vi "Stroker Wizard.vi"(1 "Stroker Wizard L1":u16, 2 "Stroker Wizard L2":u16, 11 "error in (no error)":errorcluster) -> ()   [LabVIEW 2011]
uses:
  Analog Var Disp 0 sif.ctl
  Status indicator Black Small.ctl
  Controls/Tristate/Tristate Valve state.ctl
  Controls/Slips Type Radio.ctl
  Tool/Variable List Tool Analog.ctl
  Application Structure/Options/Action GFV Settings.ctl
  Tool/Stroker/def/Tool specific commands.ctl
  Application Structure/Options/Options PageID.ctl
  Measurments Handling/Common/Variable List Common Digital.ctl
  Measurments Handling/Status Digitalish.ctl
  Tool/Variable List Tool Digital.ctl
  Application Structure/QSM State List.ctl
  emi Lib/System 01/0 - General/App/Loop control 2/Private/_emi_SMLoop Control Single.vi
  emi Lib/System 01/0 - General/App/Loop control 2/Private/_emi_ SMLoop start condition.vi
  emi Lib/System 01/0 - General/App/Loop control 2/Private/_emi_ SMLoop Error Check.vi
  emi Lib/Basic/0 - General/Error/emi_Is Error.vi
  emi Lib/System 01/0 - General/App/Loop control 2/Private/_emi_SMLoop Register new.vi
  emi Lib/System 01/0 - General/S&E reporting/emi_Send S&E Error message.vi
  emi Lib/Basic/0 - General/Error/emi_ Is Error state.vi
  emi Lib/System 01/0 - General/emi_Read System ID.vi
  emi Lib/System 01/0 - General/App/Loop control/Private/_emi_GFV Loop Running.vi
  emi Lib/System 01/0 - General/App/Loop control 2/Private/_emi_ SMLoop Restart Counter.vi
  emi Lib/System 01/0 - General/App/Loop control/Private/_emi_GFV stop a loop so it can reset.vi
  emi Lib/System 01/0 - General/App/Loop control 2/Private/_emi_ SMLoop Restart.vi
  emi Lib/System 01/0 - General/App/Loop control/Private/_emi_GFV Loop Linking.vi
  emi Lib/System 01/0 - General/App/Loop control/Private/_emi_GFV Loop Enable.vi
  emi Lib/System 01/0 - General/App/Private/_emi_GFV App Close.vi
  emi Lib/System 01/0 - General/Private/_emi_GFV System ID.vi
  emi Lib/System 01/0 - General/S&E reporting/Private/_emi_S&E Q Generator.vi
panel:
  in  "Tab Control":enum32{"Waiting", "Wizard", "Timeout"}(tab)
  out "Waiting Lights":T1
  in  "Close":bool
  in  "Size":T2=enum."338 MRS"
  out "Voltage Down Hole":T3={"Value"=nan, "Unit"="", "Status"=0} caption="Voltage Downhole(PCP)" {"Value" format="%#.1f"}
  out "St Anchor":T5 caption="Anchor"
  out "St Solonoid State Stroker":T5 caption="Direction"
  out "St Solonoid State Master":T5 caption="Stroker Enabled"
  in  "Go to default pos":bool
  out "Anchor behavior":string
  out "Stroker behavior":string
  out "Stroker force limit":string caption="tonne"
  in  "Timeout Close":bool
  # "Waiting for Telemetry to start"
  # "Stroker Wizard"
  # "Default Settings"
  # "Slips"
  # "Solenoid positions"
  # "Telemetry Timeout!"
  # "Telemetry failed to start. Voltage will be reset."
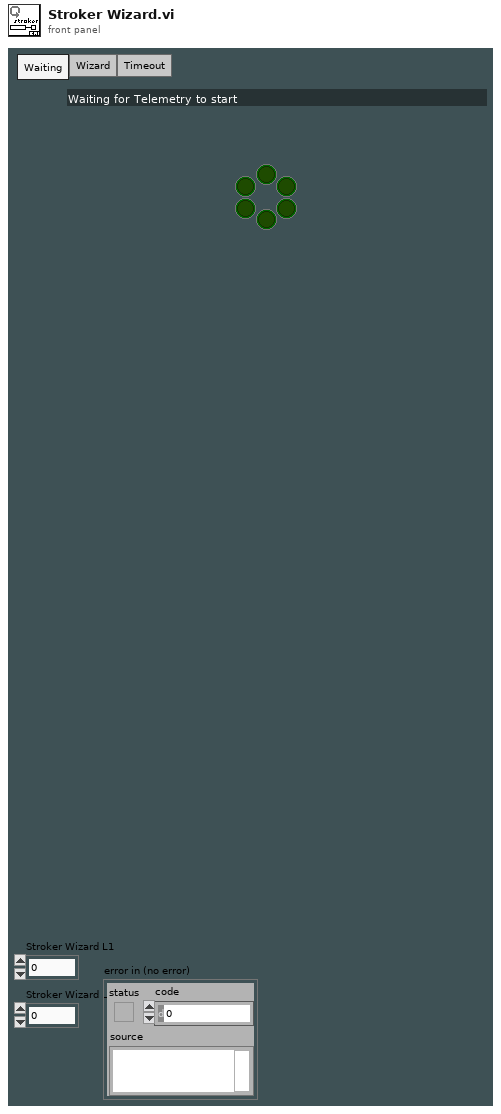
[diagram p1: front panel]
types:
  T1 = cluster{"DNL_wait 1":bool, "DNL_wait 1":bool, "DNL_wait 1":bool, "DNL_wait 1":bool, "DNL_wait 1":bool, "DNL_wait 1":bool}
  T2 = typedef "Slips Type Radio.ctl" = enum32{"No Selection", "338 MRS", "3,9 MRS"}
  T3 = typedef "Analog Var Disp 0 sif.ctl" = cluster{"Value":dbl, "Unit":string, "Status":T4}
  T4 = typedef "Status indicator Black Small.ctl" = u16
  T5 = typedef "Tristate Valve state.ctl" = u16
  T6 = typedef "Variable List Tool Digital.ctl" = enum16{"Tool Error Controller", "Tool Stopped Controller", "Tool Relay 1", "Tool Relay 2", "Tool Both Relays", "Tool node Pressure 1", "Tool Error Pressure 1", "Tool Stopped Pressure 1", "Tool node Pressure 2", "Tool Error Pressure 2", "Tool Stopped Pressure 2", "Tool node Solenoid", "Tool Error Solenoid", "Tool Stopped Solenoid", "Tool Solenoid 1", "Tool Solenoid 2", "Tool Solenoid 3", "Tool node PSU", "Tool Error PSU", "Tool Stopped PSU", "Upper Tension Sub", "Tool Error Upper Tension Sub", "Tool Stopped Upper Tension Sub", "Lower Tension Sub", "Tool Error Lower Tension Sub", "Tool Stopped Lower Tension Sub", "Stroke Target seeking", "Stroke Moving Out", "Stroke Moving Inn", "Stroke valves set for Out", "Stroke valves set for In", "Stroke In (force)", "Stroke Out (force)", "Stroke Force decreasing(in)", "Stroke Force decreasing(out)", "Stroke Force change not correct", "Stroke SLIPS established P1", "Stroke SLIPS established P2", "Stroke SLIPS established", "Stroke Pressure Monitor Ongoing", "Stroke Pressure Monitor Ending ", "Tool Stroke enable Valve", "Tool Stroke direction Valve", "Tool Anchor Valve", "Stroker Var19 - Reserved", "Stroker Var20 - Reserved", "Stroker Var21 - Reserved", "Stroker Var22 - Reserved", "Stroker Var23 - Reserved", "Stroker Var24 - Reserved", "Tractor Var1 - Reserved", "Tractor Var2 - Reserved", "Tractor Var3 - Reserved", "Tractor Var4 - Reserved", "Tractor Var5 - Reserved", "Tractor Var6 - Reserved", "Tractor Var7 - Reserved", "Tractor Var8 - Reserved", "Oil filling mode", "Mill Bit Direction", "Position control", "Anchor", "Driller Var5 - Reserved", "Driller Var6 - Reserved", "Driller Var7 - Reserved", "Driller Var8 - Reserved"}
  T7 = typedef "Status Digitalish.ctl" = enum16{"NA", "False", "True"}
  T8 = typedef "Variable List Common Digital.ctl" = enum16{"PCP Connected", "PCP PC Control", "HV PSU connected", "HV PSU HV Active", "Modem Connected", "Tool Connected", "CanBus interface"}
  T9 = typedef "QSM State List.ctl" = enum16{"Idle", "Init <<<Start>>>", "Init Reg Controlers", "Init Stroker Ref FGV", "Init Driller Ref FGV", "Init Tractor Ref FGV", "Init All loops", "Init Mem Ctls", "Init GUI", "Init<<<End>>>", "Show options", "Options updated", "Show User Dialog", "User Updated", "Show About", "Show Help", "Debug Visibility", "End Application", "Mem Ctls", "Mem Graphs", "Post", "-------------", "Dialog Common Analog", "Chart Init", "Chart Var Selector Rings init", "Chart Read Settings from INI", "Chart Clear", "Chart Selection Changed", "Chart Time Changed", "Graph Dialog Show", "Annotation, New", "Annotation Created", "PCP CMD", "Show Welcome screen", "Dialog Tool analog", "Update PCP resistance", "Tool CMD", "Chart single autoscale", "Tool connenction state", "Show detailed view", "Sequences updated", "Show stroker wizard", "Change tool", "Reset Telemetry", "Update control units", "Stop Logging", "Start New Loggfile", "Log Init", "Copy INI files"}
  T10 = enum8{"Enabled", "Disabled", "Disabled and Grayed Out"}
  T11 = typedef "Action GFV Settings.ctl" = enum16{"Init", "Get From INI", "Put In INI", "Get Settings", "Get Update Index", "Set Setting"}
  T12 = typedef "Tool specific commands.ctl" = enum16{"controller relay 1 on", "controller relay 1 off", "controller relay 2 on", "controller relay 2 off", "Solonoid 1 (master) on", "Solonoid 1 (master) off", "Solonoid 2 (Stroker) on", "Solonoid 2 (Stroker) off", "Solonoid 3 (Anchor) on", "Solonoid 3 (Anchor) off", "Controller relay 1 & 2 on", "Controller relay 1 & 2 off", "Controller relay 1 on, 2 off", "Controller relay 1 off, 2 on", "STROKER tool: Stop Force Mon", "High-G Stop", "High-G Get data", "High-G Stop Get data", "STROKER tool: Stroke out", "STROKER tool: Stroke in", "STROKER tool: Stroke stop", "STROKER tool: Stroke go to", "STROKER tool: Stop Homing", "STROKER tool: Start Force Mon dir in", "STROKER tool: Start Force Mon dir out", "Controller STOP"}
  T13 = typedef "Options PageID.ctl" = enum16{"P 1 (App)", "P 2", "P 3", "P 4", "P 5", "P 6 (Err)", "P 7 (Expert)", "P 8", "C 1", "C 2"}
  T14 = typedef "LEIN custom reply Q.ctl" = refnum<queue>
  T15 = typedef "_emi_ SMLoop sates.ctl" = enum16{"Init", "Standby", "Start", "Normal Operation", "Stop", "Error Handling", "End", "Post"}
  T16 = typedef "Variable List Tool Analog.ctl" = enum16{"Tool Max Temperature", "Tool (Controller) Temperature", "Tool Supply Voltage", "Tool (Controller) Current", "Tool Acceleration X", "Tool Acceleration Y", "Tool Acceleration Z", "Tool Acceleration Sum", "Tool Inclination", "Tool Rotation", "Tool GP Sensor 1", "Tool GP Sensor 2", "Tool (Pressure 1) Temperature", "Tool Pressure 1 RAW", "Tool (Pressure 2) Temperature", "Tool Pressure 2 RAW", "Tool (Solenoid) Temperature", "Tool Solenoid Position", "PSU Temp", "Head Voltage", "PSU Main Voltage out", "PSU Main Current out", "Upper Tension Sub Temp", "Tool Upper Tension Sub Raw", "Lower Tension Sub Temp", "Tool Lower Tension Sub Raw", "Tool Var27 - Reserved", "Tool Var28 - Reserved", "Tool Var29 - Reserved", "Tool Var30 - Reserved", "Stroke Extension", "Stroke In Force", "Stroke Out Force", "Stroke Force", "Stroker Pressure 1", "Stroker Pressure 2", "Stroker Upper Tension Sub", "Stroker Lower Tension Sub", "Stroker Var09 - Reserved", "Stroker Var10 - Reserved", "Tractor Upper Tension Sub", "Tractor Lower Tension Sub", "Tractor Var03 - Reserved", "Tractor Var04 - Reserved", "Tool Temperature sensor", "Tool Motor Voltage", "Tool Motor Current", "Tool Motor Torque", "Tool weight on bit", "Tool Motor RPM"}
  T17 = typedef "Options  All pages and custom.ctl" = cluster{"P 1 (App)":T18, "P 2":T19, "P 3":T20, "P 4":T23, "P 5":T27, "P 6 (Err)":T28, "P 7 (Expert)":T29, "P 8 (Depth)":T31, "C 1":T32, "C 2":T33}
  T18 = typedef "Options Page 1 (App).ctl" = cluster{"Result files":path, "PCP Interface":string, "Tractor/Stroker Interface":string, "Tractor Interface":string, "Modem Status Interface":string, "Audible Alarm":bool, "Force alarm on Technical":bool, "Force alarm on HH":bool, "Force alarm on LL":bool, "Force alarm on H":bool, "Force alarm on L":bool}
  T19 = typedef "Options Page 2.ctl" = cluster{"Solenoid & Relay latching time":u16, "Tractor relay 1":dbl, "Tractor relay 2":dbl, "Tractor Solenoid limit":dbl}
  T20 = typedef "Options Page 3.ctl" = cluster{"Min resistance":dbl, "Max resistance":dbl, "Head voltage range":T21, "Max voltage jump":dbl, "Maximum resistance change":dbl, "Start Telemetry Voltage":dbl, "Start Telemetry Timeout":dbl, "Start Motor Voltage":dbl, "Stop Motor Voltage":dbl, "Pass Mode Warning Voltage":dbl, "Relay Switch Voltage":dbl, "Relay Status Loss Voltage":dbl, "Samples to average":i32, "PSU type DO NOT USE":T22, "Magna OVP":dbl, "Magna Current Limit":dbl}
  T21 = typedef "PCP type List.ctl" = enum16{"0 - 350V", "0 - 450V", "0 - 600V"}
  T22 = typedef "PSU Type.ctl" = enum16{"Unipower", "Magna 8.3A", "Magna 12A", "None"}
  T23 = typedef "Options Page 4.ctl" = cluster{"Solenoid & Relay latching time":u16, "Stroker relay 1":dbl, "Stroker Relay 2":dbl, "Stroker Solenoid limit":dbl, "Force det.":T24, "Stroke force lim.":dbl, "Anchor Enabled Pressure":dbl, "Tacometer puls":dbl, "Default anchor behavior":T25, "Default stroker behavior":T26, "Default stroker force limit (tonne)":dbl, "Slips Size":T2}
  T24 = typedef "Stroke force selector.ctl" = enum16{"Stroke in = node 1", "Strok out = node 1"}
  T25 = typedef "Default anchor behavior.ctl" = enum16{"Do nothing", "Set Anchor", "Release Anchor"}
  T26 = typedef "Default stroker behavior.ctl" = enum16{"Do nothing", "Stop", "Go Out", "Go In"}
  T27 = typedef "Options Page 5.ctl" = cluster{"Solenoid & Relay latching time":u16, "Driller relay 1":dbl, "Driller Relay 2":dbl, "Driller  Solenoid limit":dbl}
  T28 = typedef "Options Page 6 (Err).ctl" = cluster{"Error and event files":path}
  T29 = typedef "Options Page 7 (Expert).ctl" = cluster{"Show Debug":bool, "Log debug messages":bool, "Additional debug messages":bool, "Start Beagle with Simulator data":bool, "Workshop mode":bool, "Modem baud":u16, "enumCANCOM":bool, "Modem sim":T30, "Telemetry Timeout Disable":i32, "Buffer size":i32, "Upd regular data":bool, "Cable comp":cluster{"VMOD1 Voltage(V)":dbl, "VMOD2 Voltage(V)":dbl}}
  T30 = typedef "Modem simulation setup.ctl" = cluster{"Modem dealay sim":bool, "Sim baud Tx":u16, "Bit Error fraction Tx":dbl, "Sim baud Rx":u16, "Bit Error fraction Rx":dbl}
  T31 = typedef "Options Page 8 (Depth).ctl" = cluster{"Winch Spool Circumference":dbl, "Winch Pulses per Revolution":dbl, "Current Depth":dbl}
  T32 = typedef "Options Custom 1.ctl" = cluster{"Depth Updated":bool, "Depth Offset":dbl}
  T33 = typedef "Options Custom 2.ctl" = cluster{"Placeholder":bool}
  T34 = typedef "Fixed Analog Channel Definition.ctl" = cluster{"ID":u16, "Name":string, "Quantity":T35, "Unit":string, "Maximum upd":T36, "Comment":string, "Help file Name":string, "Help file Section ":string, "Category":T37, "User adjustable Scaling":bool, "Default Scaling":T38, "Default Unit":i32, "Classification":T39}
  T35 = typedef "Quantity enum.ctl" = enum16{"NA", "Acceleration", "Angle", "Current", "Force", "Distance", "Pressure", "Resistance", "Rotational Speed", "Speed", "Temperature", "Tension", "Torque", "Voltage", "Weight"}
  T36 = typedef "Update frequensies.ctl" = enum16{"2 Hz", "1 Hz", "0.1 Hz"}
  T37 = typedef "Channel catagory Enum.ctl" = enum16{"No Category", "Power", "Temperature", "Pressure"}
  T38 = typedef "Scaling.ctl" = cluster{"Gain":dbl, "Offset":dbl}
  T39 = typedef "Channel Classification Enum.ctl" = enum16{"Basic", "Advanced", "Expert", "Unused"}
  T40 = typedef "User Setting Analog Channel Bg.ctl" = cluster{"Scaling":T38, "Limits and responces":T41, "Allow Graph selection by user":bool, "Unit":u16}
  T41 = typedef "Alarm Setup Analog.ctl" = cluster{"Technical Error(NA)":T42, "LL":T42, "L":T42, "H":T42, "HH":T42, "Limits":T44}
  T42 = typedef "Alarm Responce.ctl" = cluster{"Action":T43, "Alarm":bool}
  T43 = typedef "Action List.ctl" = enum16{"No Action", "Stop Motor", "Turn Off HV"}
  T44 = typedef "Limits.ctl" = cluster{"LL":dbl, "L":dbl, "H":dbl, "HH":dbl}
  T45 = cluster{"Placeholder":bool, "Timer value":timestamp, "Timed out":bool, "Waiting lights":bool[], "Tool Connected":bool}
  T46 = typedef "List of tools.ctl" = enum16{"Stroker", "Driller", "Tractor"}
  T47 = cluster{"[0]":bool, "[1]":bool, "[2]":bool, "[3]":bool, "[4]":bool, "[5]":bool}
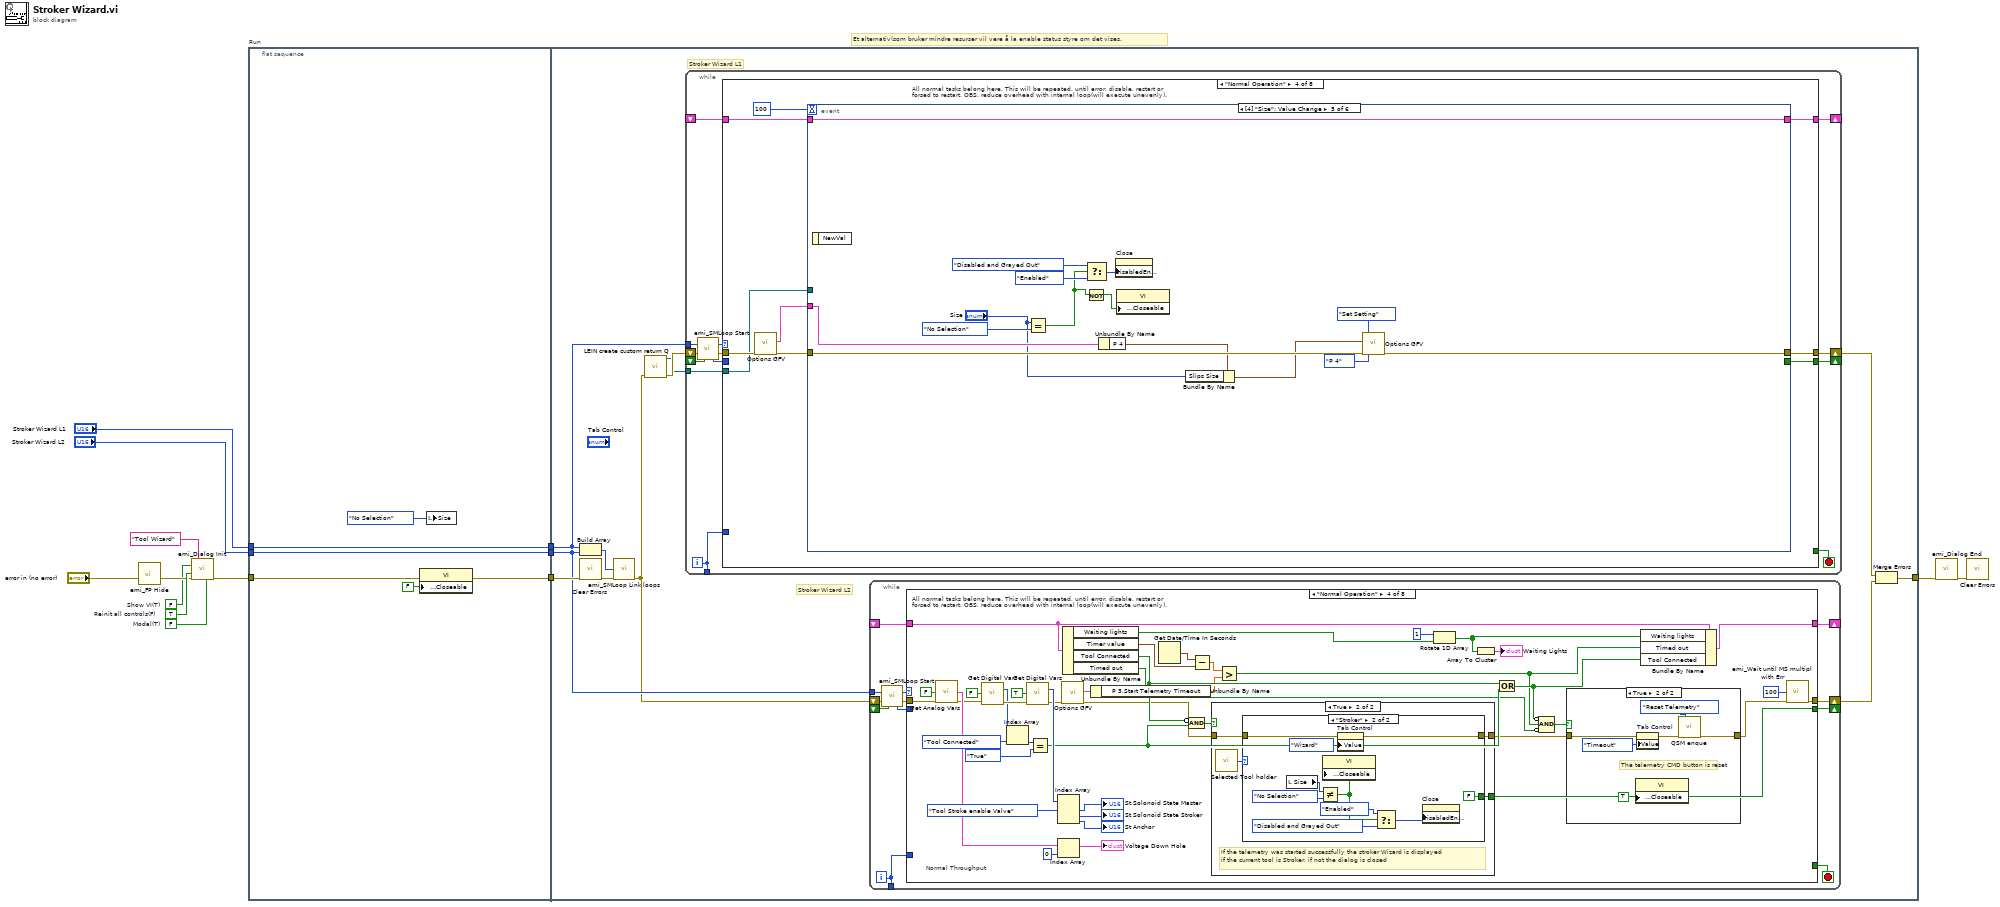
[diagram p0: block diagram]
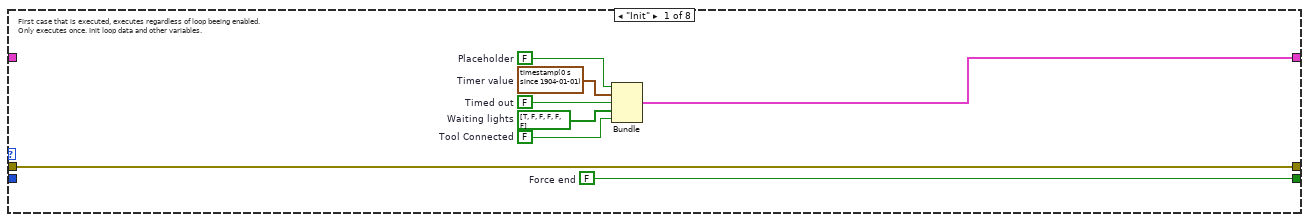
[diagram p2: hidden frame]
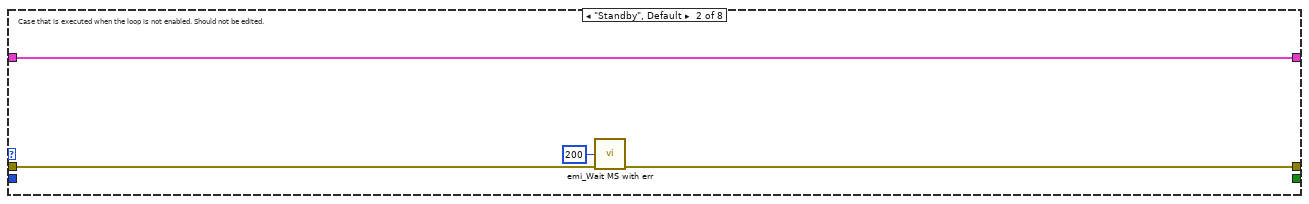
[diagram p3: hidden frame]
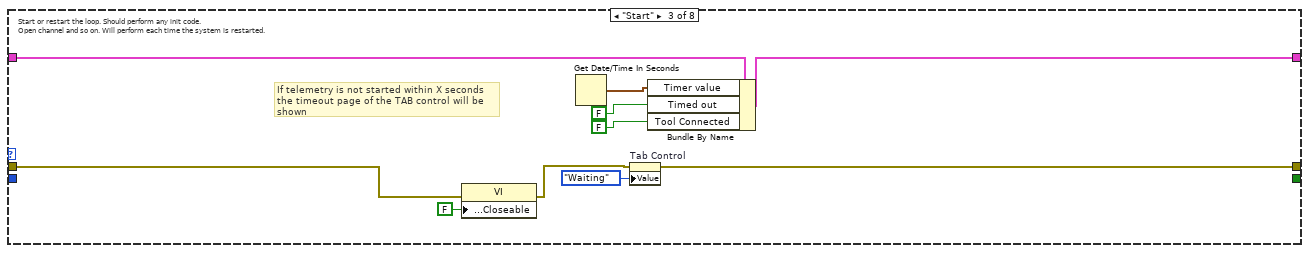
[diagram p4: hidden frame]
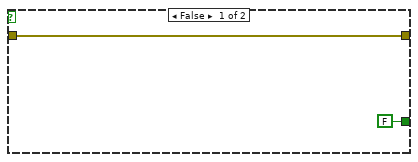
[diagram p6: hidden frame]
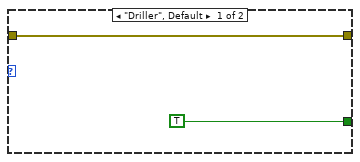
[diagram p7: hidden frame]
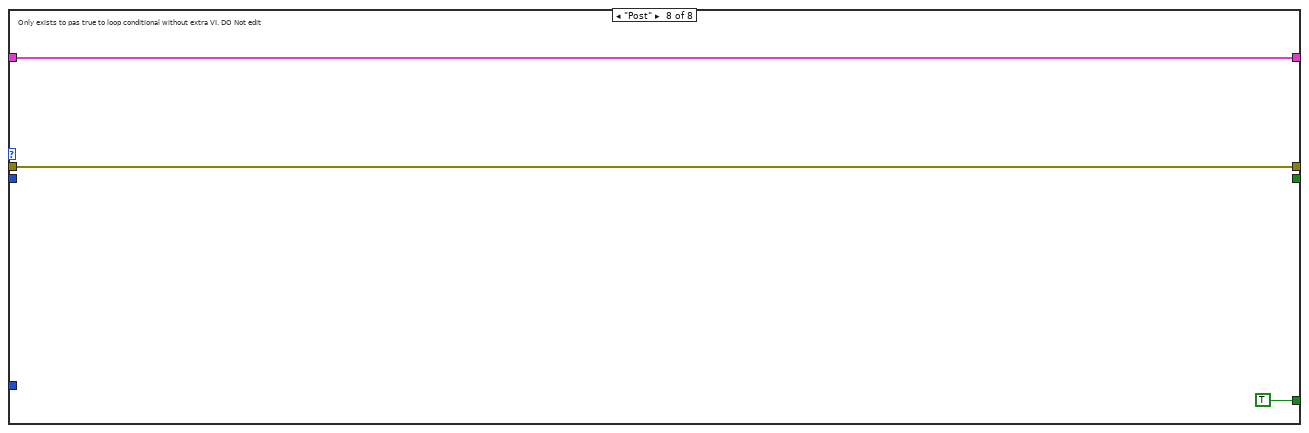
[diagram p11: hidden frame]
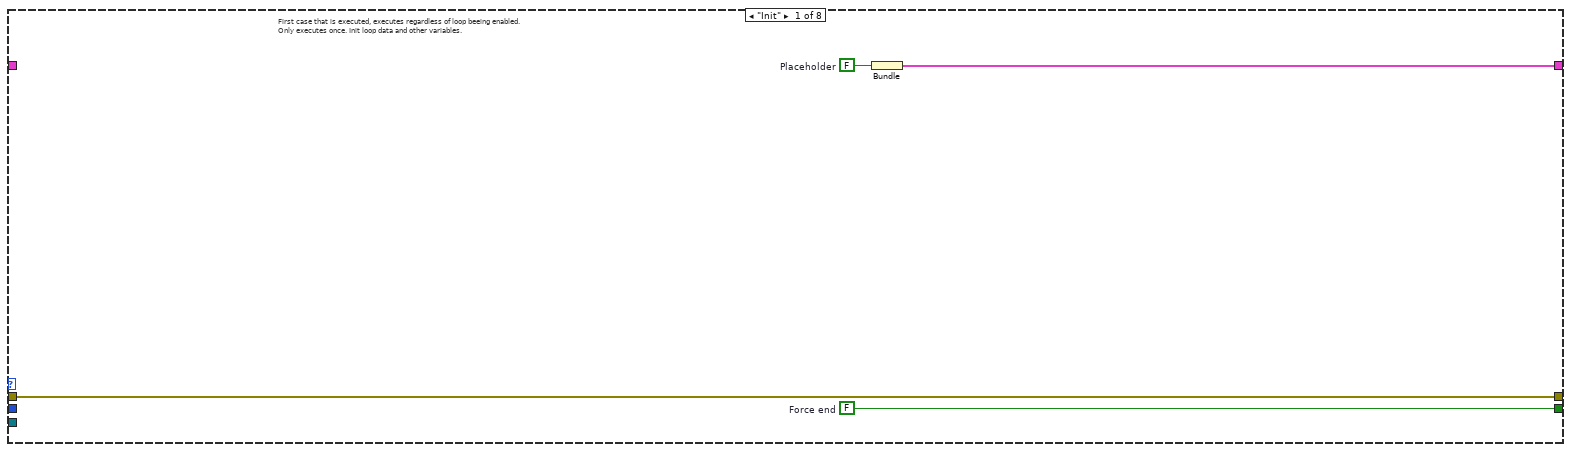
[diagram p12: hidden frame]
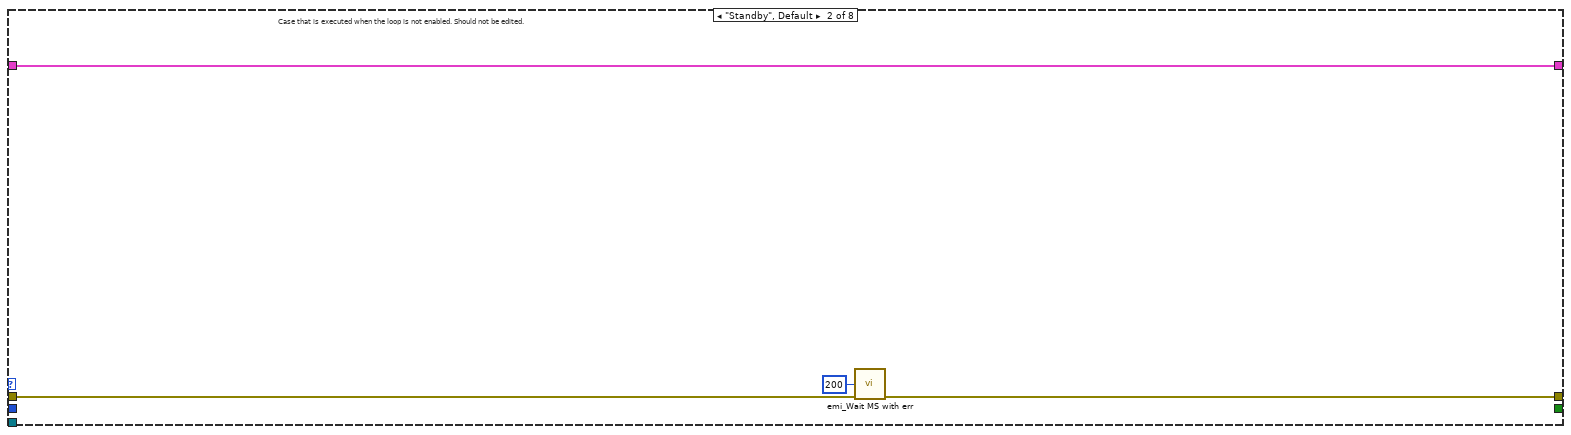
[diagram p13: hidden frame]
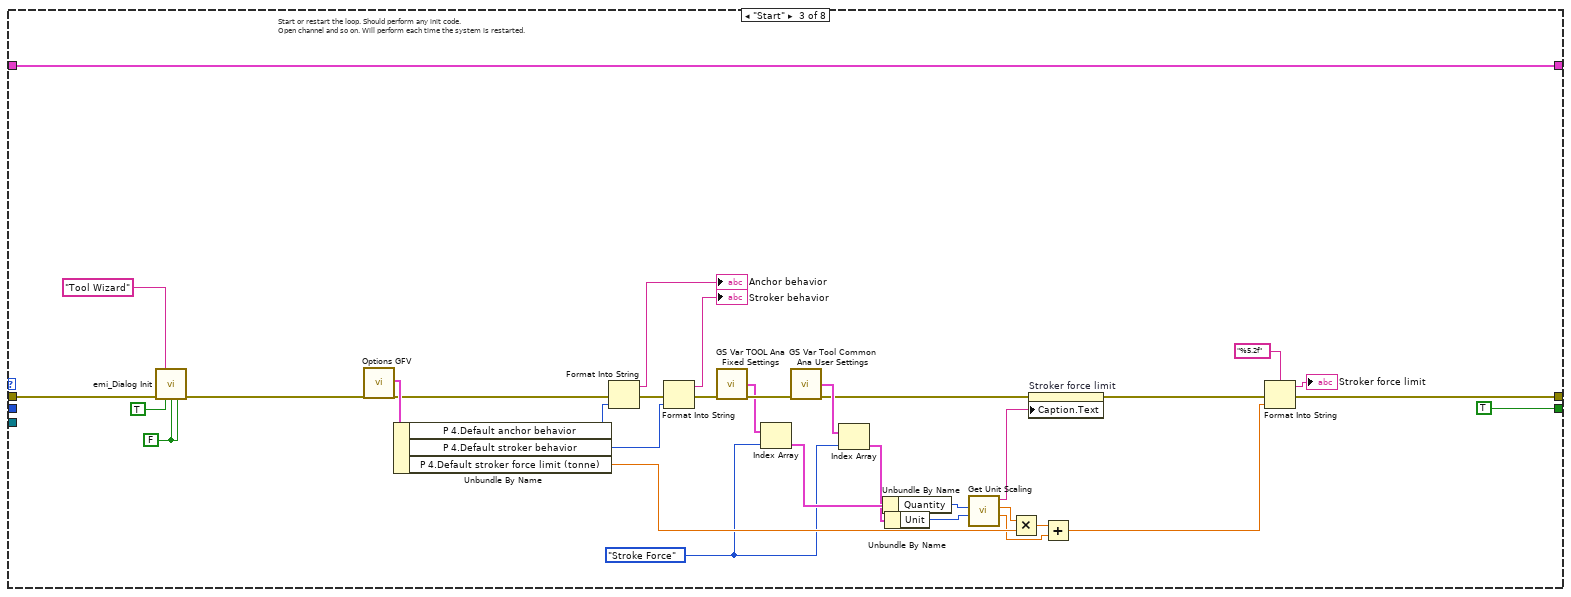
[diagram p14: hidden frame]
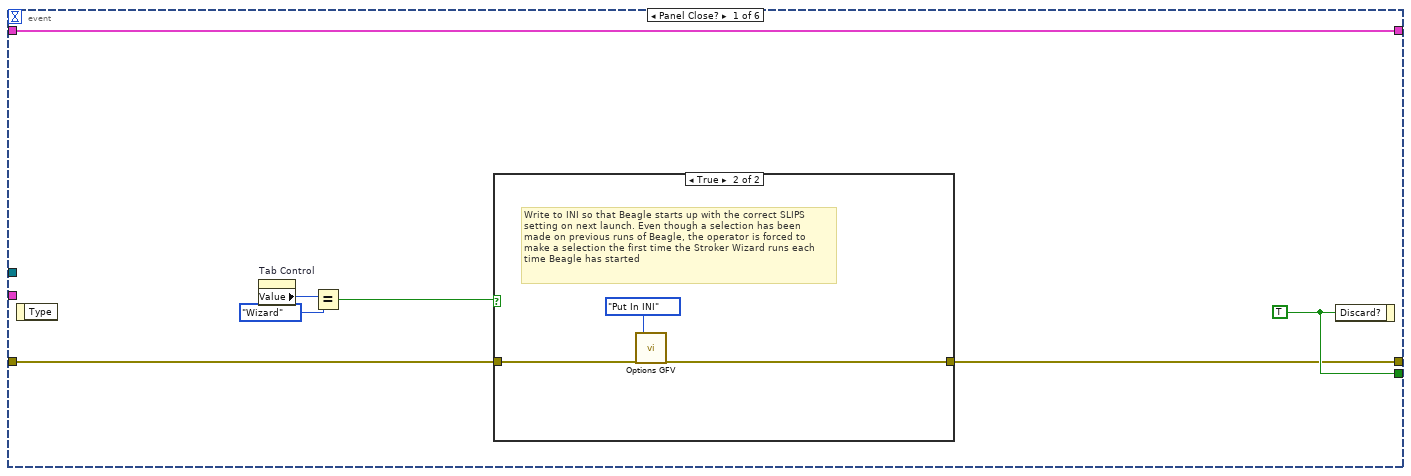
[diagram p15: hidden frame]
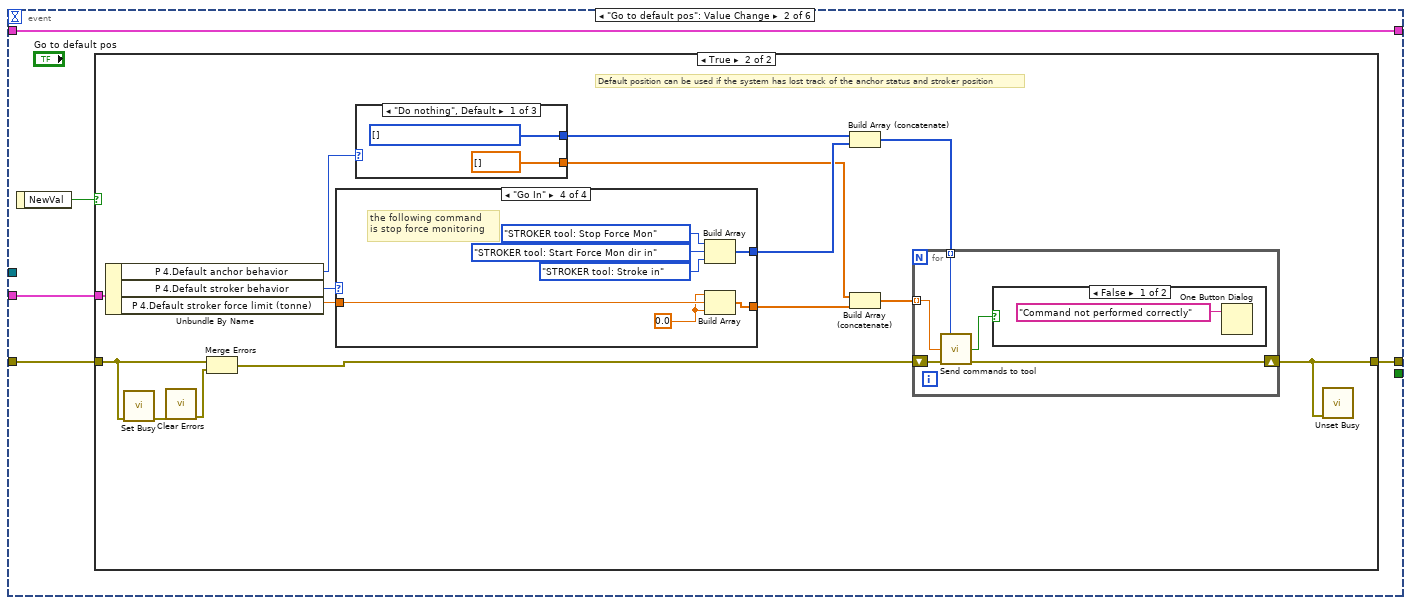
[diagram p17: hidden frame]
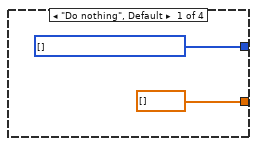
[diagram p20: hidden frame]
diagram:
  w10 = FALSE  # Show VI(T)
  w12 = TRUE  # Reinit all controls(F)
  w13 = FALSE  # Modal(T)
  # "Et alternativ(som bruker mindre resurser vil vere å la enable status styre om det vises."
  n1 = call "emi_FP Hide.vi"("error in (no error)"="error in (no error)") -> ("error out"=w11:errorcluster)  [unwired: 13 in, 1 out]
  n2 = call "emi_Dialog Init.vi"("Header String(\"\")"="Tool Wizard" ("Header String(\"\")"), "Show VI(T)"=w10, "Reinit all controls(F)"=w12, "error in"=w11, "Modal(T)"=w13) -> ("error out"=w4:errorcluster)  [unwired: 10 in]
  n3 = flat-sequence "Run" {
    tunnel: "Stroker Wizard L2" -> [w19]
    tunnel: "Stroker Wizard L1" -> [w20]
    tunnel: w4 -> [w18]
    tunnel: [w17] -> w3
    tunnel: [w20] -> w2
    tunnel: [w19] -> w1
    tunnel: [w28] -> w9
    tunnel: w3 -> [w31]
    tunnel: w2 -> [w26]
    tunnel: w1 -> [w25]
    frame #0 {
      n4 = property on="Property Node" class="VI"(error in=w18, "Front Panel.Closeable"=FALSE ("Front Panel Window:Closeable")) -> (error out=w17:errorcluster)  [unwired: 1 in, 1 out]
      n5 = local write "Size"(Slips_Type_Radio."No Selection" ("Size")) -> ()
    }
    frame #1 {
      # "Stroker Wizard L2"
      # "Stroker Wizard L1"
      n6 = Build Array(w26, w25) -> (w24:u16[])
      n7 = call <vilib>:"Clear Errors.vi"("error in (no error)"=w31) -> ("error out"=w27:errorcluster)  [unwired: 6 in]
      n8 = call "emi_SMLoop Link loops.vi"("Loop IDS"=w24, "error in (no error)"=w27) -> ("error out"=w23:errorcluster)  [unwired: 13 in]
      n9 = call "LEIN create custom return Q.vi"("error in (no error)"=w23) -> ("LEIN custom reply Q"=w21:T14, "error out"=w22:errorcluster)  [unwired: 13 in]
      n10 = while {
        shift-right: [w155] -> _
        shift-left: _ -> [w152]
        shift-right: [w153] -> w30
        shift-left: w22 -> [w150]
        tunnel: [w143] -> _
        shift-right: [w151] -> _
        shift-left: _ -> [w146]
        tunnel: w26 -> [w147]
        tunnel: w21 -> [w144]
        i -> [w143]
        stop <- w154 stop-if-true
        n11 = call "emi_SMLoop Start.vi"("Loop ID"=w147, "error in (no error)"=w150, "Force Stop(F)"=w146) -> ("Loop command"=w148:T15, "error out"=w149:errorcluster, "Loop ID out"=w145:i32)  [unwired: 10 in]
        n12 = case shown="\"Normal Operation\"" w148 {
          tunnel: [w158 w160 w197 w204 w309 w324 w325 w328] -> w155
          tunnel: [_ _ _ _ _ _ _ TRUE] -> w154
          tunnel: w149 -> [w159 w162 w196 w206 w308 w323 w326 w329]
          tunnel: [w159 w161 w171 w205 w304 w323 w326 w329] -> w153
          tunnel: w152 -> [_ w160 w197 w203 w309 w324 w325 w328]
          tunnel: [w156 _ TRUE ("Discard?") w202 _ _ _ _] -> w151
          tunnel: w145 -> [_ _ _ _ w307 _ _ _]
          tunnel: w144 -> [_ _ _ w201 _ _ _ _]
          tunnel: w143 -> [_ _ _ _ _ _ _ _]
          frame "Init" {
            w156 = FALSE  # Force end
            w157 = FALSE  # Placeholder
            # "First case that is executed, executes regardless of loop beeing enabled.\nOnly executes once. Init loop data and other variables."
            n13 = Bundle("Placeholder"=w157) -> (w158:cluster{"Placeholder":bool})  [unwired: 1 in]
          }
          frame "Standby", Default {
            # "Case that is executed when the loop is not enabled. Should not be edited."
            n14 = call "emi_Wait MS with err.vi"("milliseconds to wait(0)"=u32 200, "error in (no error)"=w162) -> ("error out"=w161:errorcluster)  [unwired: 13 in]
          }
          frame "Start" {
            w165 = Variable_List_Tool_Analog."Stroke Force" ("Variable ID")
            w193 = FALSE ("Set BG Color(T)")
            # "Start or restart the loop. Should perform any init code. \nOpen channel and so on. Will perform each time the system is restarted."
            n15 = call "emi_Dialog Init.vi"("Header String(\"\")"="Tool Wizard" ("Header String(\"\")"), "error in"=w196, "Center in bottom FP(T)"=TRUE, "Set BG Color(T)"=w193, "Modal(T)"=w193) -> ("error out"=w164:errorcluster)  [unwired: 10 in]
            n16 = call "Options GFV.vi"("error in (no error)"=w164) -> ("Options"=w191:T17, "error out"=w190:errorcluster)  [unwired: 16 in, 1 out]
            n17 = Unbundle By Name(w191) -> ("P 4.Default anchor behavior"=w188:T25, "P 4.Default stroker behavior"=w187:T26, "P 4.Default stroker force limit (tonne)"=w169:dbl)
            n18 = Format Into String(error in=w190, w188) -> (resulting string=→"Anchor behavior":string, error out=w189:errorcluster)  [unwired: 2 in]
            n19 = Format Into String(error in=w189, w187) -> (resulting string=→"Stroker behavior":string, error out=w174:errorcluster)  [unwired: 2 in]
            n20 = call "GS Var TOOL Ana Fixed Settings.vi"("error in (no error)"=w174) -> ("Tool Analog var Fixed out"=w177:T34[], "error out"=w182:errorcluster)  [unwired: 12 in, 1 out]
            n21 = Index Array(array=w177, index=w165) -> (element=w179:T34)
            n22 = call "GS Var Tool Common Ana User Settings.vi"("error in (no error)"=w182) -> ("Tool Analog var User settigns out"=w176:T40[], "error out"=w173:errorcluster)  [unwired: 12 in, 1 out]
            n23 = Index Array(array=w176, index=w165) -> (element=w178:T40)
            n24 = Unbundle By Name(w179) -> ("Quantity"=w180:T35)
            n25 = Unbundle By Name(w178) -> ("Unit"=w181:u16)
            n26 = call "Get Unit Scaling.vi"("Unit Index"=w181, "Quantity"=w180) -> ("Offset"=w167:dbl, "Gain"=w170:dbl, "Unit"=w175:string)  [unwired: 7 in]
            n27 = Multiply(x=w170, y=w169) -> (x*y=w168:dbl)
            n28 = property on="Stroker force limit" class="Str"(error in=w173, "Caption.Text"=w175) -> (error out=w172:errorcluster)  [unwired: 1 in, 1 out]
            n29 = Add(x=w168, y=w167) -> (x+y=w166:dbl)
            n30 = Format Into String(format string="%5.2f", error in=w172, w166) -> (resulting string=→"Stroker force limit":string, error out=w171:errorcluster)  [unwired: 1 in]
          }
          frame "Normal Operation" {
            # "All normal tasks belong here. This will be repeated, until error, disable, restart or\nforsed to restart. OBS, reduce overhead with internal loop(will execute unevenly)."
            n31 = call "Options GFV.vi"("error in (no error)"=w206) -> ("Options"=w198:T17, "error out"=w199:errorcluster)  [unwired: 16 in, 1 out]
            n32 = event shown="[4] \"Size\": Value Change" {
              selector: _ -> [_ _ _ _ _ _]
              dyn-events: _ -> [_ _ _ _ _ _]
              timeout: 100 -> [_ _ _ _ _ _]
              tunnel: w199 -> [w211 w221 w278 w285 w296 w302]
              tunnel: w203 -> [w213 w222 w279 w286 w301 w303]
              tunnel: [w213 w222 w279 w286 w301 w303] -> w204
              tunnel: [w210 w219 w276 w285 w295 w302] -> w205
              tunnel: [w212 _ w277 w284 _ _] -> w202
              tunnel: w201 -> [_ _ _ _ _ _]
              tunnel: w198 -> [_ w218 _ _ w293 _]
              event Panel Close? {
                w212 = TRUE ("Discard?")
                n33 = event-data() -> ()  [unwired: 1 in, 1 out]
                n34 = property on="Tab Control" class="TabCtl (strict)"() -> ("Value"=w209:enum32{"Waiting", "Wizard", "Timeout"})  [unwired: 2 in, 2 out]
                n35 = Equal?(x=w209, y=enum32{"Waiting", "Wizard", "Timeout"}."Wizard") -> (x = y?=w207:bool)
                n36 = case shown="True" w207 {
                  tunnel: w211 -> [w214 w216]
                  tunnel: [w214 w215] -> w210
                  frame False {
                  }
                  frame True {
                    # "Write to INI so that Beagle starts up with the correct SLIPS \nsetting on next launch. Even though a selection has been\nmade on previous runs of Beagle, the operator is forced to\nmake a selection the first time the Stroker Wizard runs each\ntime Beagle has started"
                    n37 = call "Options GFV.vi"("error in (no error)"=w216, "Action(Get Settings)"=Action_GFV_Settings."Put In INI") -> ("error out"=w215:errorcluster)  [unwired: 15 in, 2 out]
                  }
                }
                n38 = event-data("Discard?"=w212) -> ()  [unwired: 1 in, 1 out]
              }
              event "Go to default pos": Value Change {
                n39 = event-data() -> ("NewVal"=w220:bool)  [unwired: 1 in]
                n40 = case shown="True" w220 {
                  tunnel: [w223 w225] -> w219
                  tunnel: w221 -> [w223 w236]
                  tunnel: w218 -> [_ w235]
                  frame False {
                  }
                  frame True {
                    # "Default position can be used if the system has lost track of the anchor status and stroker position"
                    n41 = Unbundle By Name(w235) -> ("P 4.Default anchor behavior"=w224:T25, "P 4.Default stroker behavior"=w234:T26, "P 4.Default stroker force limit (tonne)"=w233:dbl)
                    n42 = call <vilib>:"Set Busy.vi"("error in (no error)"=w236) -> ("error out"=w237:errorcluster)  [unwired: 9 in, 1 out]
                    n43 = call <vilib>:"Clear Errors.vi"("error in (no error)"=w237) -> ("error out"=w238:errorcluster)  [unwired: 6 in]
                    n44 = Merge Errors(w236, w238) -> (w232:errorcluster)
                    n45 = case shown="\"Go In\"" w234 {
                      tunnel: w233 -> [_ _ w254 w261]
                      tunnel: [w246 w251 w258 w265] -> w230
                      tunnel: [dbl[] [] w250 w257 w264] -> w228
                      frame "Do nothing", Default {
                        w246 = T12[] [] items=["controller relay 1 on", "controller relay 1 off", "controller relay 2 on", "controller relay 2 off", "Solonoid 1 (master) on", "Solonoid 1 (master) off", "Solonoid 2 (Stroker) on", "Solonoid 2 (Stroker) off", "Solonoid 3 (Anchor) on", "Solonoid 3 (Anchor) off", "Controller relay 1 & 2 on", "Controller relay 1 & 2 off", "Controller relay 1 on, 2 off", "Controller relay 1 off, 2 on", "STROKER tool: Stop Force Mon", "High-G Stop", "High-G Get data", "High-G Stop Get data", "STROKER tool: Stroke out", "STROKER tool: Stroke in", "STROKER tool: Stroke stop", "STROKER tool: Stroke go to", "STROKER tool: Stop Homing", "STROKER tool: Start Force Mon dir in", "STROKER tool: Start Force Mon dir out", "Controller STOP"]
                      }
                      frame "Stop" {
                        w247 = 0.0 ("element")
                        # "Send both commands because we don't know\nif stroker is Homing or running in or out"
                        n46 = Build Array(Tool_specific_commands."STROKER tool: Stop Homing" ("Tool command"), Tool_specific_commands."STROKER tool: Stroke stop" ("Tool command")) -> (w251:T12[])
                        n47 = Build Array(w247, w247) -> (w250:dbl[])
                      }
                      frame "Go Out" {
                        w252 = 0.0 ("element")
                        # "the following command\nis stop force monitoring"
                        n48 = Build Array(Tool_specific_commands."STROKER tool: Stop Force Mon" ("Tool command"), Tool_specific_commands."STROKER tool: Start Force Mon dir out" ("Tool command"), Tool_specific_commands."STROKER tool: Stroke out" ("Tool command")) -> (w258:T12[])
                        n49 = Build Array(w252, w254, w252) -> (w257:dbl[])
                      }
                      frame "Go In" {
                        w260 = 0.0 ("element")
                        # "the following command\nis stop force monitoring"
                        n50 = Build Array(Tool_specific_commands."STROKER tool: Stop Force Mon" ("Tool command"), Tool_specific_commands."STROKER tool: Start Force Mon dir in" ("Tool command"), Tool_specific_commands."STROKER tool: Stroke in" ("Tool command")) -> (w265:T12[])
                        n51 = Build Array(w260, w261, w260) -> (w264:dbl[])
                      }
                    }
                    n52 = case shown="\"Do nothing\", Default" w224 {
                      tunnel: [w267 w270 w274] -> w231
                      tunnel: [dbl[] [] w268 w272] -> w226
                      frame "Do nothing", Default {
                        w267 = T12[] [] items=["controller relay 1 on", "controller relay 1 off", "controller relay 2 on", "controller relay 2 off", "Solonoid 1 (master) on", "Solonoid 1 (master) off", "Solonoid 2 (Stroker) on", "Solonoid 2 (Stroker) off", "Solonoid 3 (Anchor) on", "Solonoid 3 (Anchor) off", "Controller relay 1 & 2 on", "Controller relay 1 & 2 off", "Controller relay 1 on, 2 off", "Controller relay 1 off, 2 on", "STROKER tool: Stop Force Mon", "High-G Stop", "High-G Get data", "High-G Stop Get data", "STROKER tool: Stroke out", "STROKER tool: Stroke in", "STROKER tool: Stroke stop", "STROKER tool: Stroke go to", "STROKER tool: Stop Homing", "STROKER tool: Start Force Mon dir in", "STROKER tool: Start Force Mon dir out", "Controller STOP"]
                      }
                      frame "Set Anchor" {
                        n53 = Build Array(Tool_specific_commands."Solonoid 3 (Anchor) on" ("Tool command")) -> (w270:T12[])
                        n54 = Build Array(0.0 ("element")) -> (w268:dbl[])
                      }
                      frame "Release Anchor" {
                        n55 = Build Array(Tool_specific_commands."Solonoid 3 (Anchor) off" ("Tool command")) -> (w274:T12[])
                        n56 = Build Array(0.0 ("element")) -> (w272:dbl[])
                      }
                    }
                    n57 = Build Array (concatenate)(w231, w230) -> (w229:T12[])
                    n58 = Build Array (concatenate)(w226, w228) -> (w227:dbl[])
                    n59 = for {
                      shift-right: [w241] -> w225
                      shift-left: w232 -> [w242]
                      tunnel: w229 -> [w240] mode=indexing
                      tunnel: w227 -> [w239] mode=indexing
                      n60 = call "Send commands to tool.vi"("Tool command"=w240, "Input Data"=w239, "error in"=w242) -> ("OK"=w243:bool, "error out"=w241:errorcluster)  [unwired: 11 in]
                      n61 = case shown="False" w243 {
                        frame False {
                          n62 = One Button Dialog(message="Command not performed correctly") -> ()  [unwired: 1 in, 1 out]
                        }
                        frame True {
                        }
                      }
                    }
                    n63 = call <vilib>:"Unset Busy.vi"("error in (no error)"=w225) -> ()  [unwired: 10 in, 1 out]
                  }
                }
              }
              event "Close": Value Change {
                n64 = event-data() -> ("NewVal"=w277:bool)  [unwired: 1 in]
                n65 = case shown="True" w277 {
                  tunnel: w278 -> [w280 w283]
                  tunnel: [w280 w282] -> w276
                  frame False {
                  }
                  frame True {
                    # "Write to INI so that Beagle starts up with the correct SLIPS \nsetting on next launch. Even though a selection has been\nmade on previous runs of Beagle, the operator is forced to\nmake a selection the first time the Stroker Wizard runs each\ntime Beagle has started"
                    n66 = call "Options GFV.vi"("error in (no error)"=w283, "Action(Get Settings)"=Action_GFV_Settings."Put In INI") -> ("error out"=w282:errorcluster)  [unwired: 15 in, 2 out]
                  }
                }
              }
              event "Timeout Close": Value Change {
                n67 = event-data() -> ("NewVal"=w284:bool)  [unwired: 1 in]
              }
              event Value Change {
                n68 = event-data() -> ()  [unwired: 1 in, 1 out]
                n69 = Equal?(x="Size", y=Slips_Type_Radio."No Selection" ("Size")) -> (x = y?=w288:bool)
                n70 = Not(x=w288) -> (.not. x?=w287:bool)
                n71 = Select(t=T10."Disabled and Grayed Out" ("Disabled"), s=w288, f=T10."Enabled") -> (s? t:f=w299:T10)
                n72 = Unbundle By Name(w293) -> ("P 4"=w291:T23)
                n73 = property on="Close" class="Bool (strict)"("DisabledEnum"=w299) -> ()  [unwired: 2 in, 2 out]
                n74 = property on="Property Node" class="VI"("Front Panel.Closeable"=w287) -> ()  [unwired: 2 in, 2 out]
                n75 = Bundle By Name(cluster=w291, "Slips Size"="Size") -> (w290:T23)
                n76 = call "Options GFV.vi"("Anything"=w290, "error in (no error)"=w296, "Action(Get Settings)"=Action_GFV_Settings."Set Setting", "Setting ID"=Options_PageID."P 4") -> ("error out"=w295:errorcluster)  [unwired: 13 in, 2 out]
              }
              event Timeout {
                n77 = event-data() -> ()  [unwired: 1 in, 2 out]
              }
            }
          }
          frame "Stop" {
            # "Så ikke auto starter igjen om enablet"
            # "To alow VI to exit befor \nAplicatin End.\nFor use in dialogs"
            # "Stop the loop. May be restarted later. Close interfaces and the like"
            n78 = disable-structure shown="Enabled" {
              disable-tunnel: w308 -> [w321 w322]
              disable-tunnel: w307 -> [w320 _]
              disable-tunnel: [w318 w322] -> w306
              frame Enabled {
                n79 = call-poly "emi_SMLoop Control.vi"("Loop ID in"=w320, "Enable"=FALSE, "error in (no error)"=w321) -> ("error out"=w318:errorcluster)  [unwired: 11 in, 1 out]
              }
              frame Disabled {
              }
            }
            n80 = call "emi_FP Hide.vi"("error in (no error)"=w306) -> ("error out"=w305:errorcluster)  [unwired: 13 in, 1 out]
            n81 = disable-structure shown="Disabled" {
              disable-tunnel: w305 -> [w311 w317]
              disable-tunnel: [w310 w317] -> w304
              frame Disabled {
                n82 = call "emi_Get Debug Aditional status.vi"("error in (no error)"=w311) -> ("Debug Additional"=w313:bool, "error out"=w316:errorcluster)  [unwired: 13 in]
                n83 = call "emi_Get Debug Log status.vi"("error in (no error)"=w316) -> ("Debug Log"=w314:bool, "error out"=w315:errorcluster)  [unwired: 13 in]
                n84 = call "emi_Set Debug status.vi"("Debug Disp"=FALSE, "Debug Log"=w314, "Debug Aditional"=w313, "error in (no error)"=w315) -> ("error out"=w310:errorcluster)  [unwired: 11 in]
              }
              frame Enabled {
              }
            }
          }
          frame "Error Handling" {
            # "Loop automaticaly returns here after error is found. If error is cleared, \nLoop wil continue as normal(if was operative when error."
          }
          frame "End" {
            # "Only executes at application end has. Should performa any action the loop \nneeds to finnish. Executes only once."
          }
          frame "Post" {
            # "Only exists to pas true to loop conditional without extra VI. DO Not edit"
          }
        }
      }
      n85 = while {
        shift-right: [w43] -> _
        shift-left: _ -> [w40]
        shift-right: [w41] -> w29
        shift-left: w23 -> [w38]
        tunnel: [w32] -> _
        shift-right: [w39] -> _
        shift-left: _ -> [w34]
        tunnel: w25 -> [w35]
        i -> [w32]
        stop <- w42 stop-if-true
        n86 = call "emi_SMLoop Start.vi"("Loop ID"=w35, "error in (no error)"=w38, "Force Stop(F)"=w34) -> ("Loop command"=w36:T15, "error out"=w37:errorcluster, "Loop ID out"=w33:i32)  [unwired: 10 in]
        n87 = case shown="\"Normal Operation\"" w36 {
          tunnel: [w51 w52 w63 w106 w134 w137 w138 w141] -> w43
          tunnel: [_ _ _ _ _ _ _ TRUE] -> w42
          tunnel: w37 -> [w49 w54 w57 w108 w135 w136 w139 w142]
          tunnel: [w49 w53 w61 w107 w135 w136 w139 w142] -> w41
          tunnel: w40 -> [_ w52 w65 w105 w134 w137 w138 w141]
          tunnel: [w50 _ _ w66 _ _ _ _] -> w39
          tunnel: w33 -> [_ _ _ _ _ _ _ _]
          tunnel: w32 -> [_ _ _ _ _ _ _ _]
          frame "Init" {
            w44 = FALSE  # Tool Connected
            w45 = FALSE  # Timed out
            w47 = FALSE  # Placeholder
            w46 = bool[] [TRUE, FALSE, FALSE, FALSE, FALSE, FALSE]  # Waiting lights
            w48 = timestamp(0 s since 1904-01-01)  # Timer value
            w50 = FALSE  # Force end
            # "First case that is executed, executes regardless of loop beeing enabled.\nOnly executes once. Init loop data and other variables."
            n88 = Bundle("Placeholder"=w47, "Timer value"=w48, "Timed out"=w45, "Waiting lights"=w46, "Tool Connected"=w44) -> (w51:T45)  [unwired: 1 in]
          }
          frame "Standby", Default {
            # "Case that is executed when the loop is not enabled. Should not be edited."
            n89 = call "emi_Wait MS with err.vi"("milliseconds to wait(0)"=u32 200, "error in (no error)"=w54) -> ("error out"=w53:errorcluster)  [unwired: 13 in]
          }
          frame "Start" {
            # "If telemetry is not started within X seconds\nthe timeout page of the TAB control will be shown"
            # "Start or restart the loop. Should perform any init code. \nOpen channel and so on. Will perform each time the system is restarted."
            n90 = property on="Property Node" class="VI"(error in=w57, "Front Panel.Closeable"=FALSE ("Front Panel Window:Closeable")) -> (error out=w56:errorcluster)  [unwired: 1 in, 1 out]
            n91 = Get Date/Time In Seconds() -> (seconds since 1Jan1904=w64:timestamp)
            n92 = property on="Tab Control" class="TabCtl (strict)"(error in=w56, "Value"=enum32{"Waiting", "Wizard", "Timeout"}."Waiting" ("Tab Control")) -> (error out=w61:errorcluster)  [unwired: 1 in, 1 out]
            n93 = Bundle By Name(cluster=w65, "Timer value"=w64, "Timed out"=FALSE, "Tool Connected"=FALSE) -> (w63:T45)
          }
          frame "Normal Operation" {
            # "Normal Throughput"
            # "All normal tasks belong here. This will be repeated, until error, disable, restart or\nforsed to restart. OBS, reduce overhead with internal loop(will execute unevenly)."
            n94 = call "Get Analog Vars.vi"("Tool"=FALSE, "error in (no error)"=w108) -> ("Analog Vars"=w94:T3[], "error out"=w72:errorcluster)  [unwired: 7 in, 5 out]
            n95 = call "Get Digital Vars.vi"("Tool"=FALSE, "error in (no error)"=w72) -> ("Values"=w92:T7[], "error out"=w101:errorcluster)  [unwired: 7 in, 5 out]
            n96 = Index Array(array=w92, index=Variable_List_Common_Digital."Tool Connected" ("Action")) -> (element=w90:T7)
            n97 = call "Get Digital Vars.vi"("Tool"=TRUE, "error in (no error)"=w101) -> ("Values"=w99:T7[], "error out"=w71:errorcluster)  [unwired: 7 in, 5 out]
            n98 = Equal?(x=w90, y=Status_Digitalish."True" ("element")) -> (x = y?=w80:bool)
            n99 = Index Array(array=w99, index #1=Variable_List_Tool_Digital."Tool Stroke enable Valve") -> (element #1=→"St Solonoid State Master":T7, element #2=→"St Solonoid State Stroker":T7, element #3=→"St Anchor":T7)  [unwired: 2 in]
            n100 = Index Array(array=w94, index=0) -> (element=→"Voltage Down Hole":T3)
            n101 = call "Options GFV.vi"("error in (no error)"=w71) -> ("Options"=w74:T17, "error out"=w70:errorcluster)  [unwired: 16 in, 1 out]
            n102 = Unbundle By Name(w105) -> ("Waiting lights"=w82:bool[], "Timer value"=w87:timestamp, "Tool Connected"=w81:bool, "Timed out"=w75:bool)
            n103 = Unbundle By Name(w74) -> ("P 3.Start Telemetry Timeout"=w73:dbl)
            n104 = Get Date/Time In Seconds() -> (seconds since 1Jan1904=w88:timestamp)
            n105 = Compound Arithmetic op=AND(invert w81, w80) -> (w79:bool)
            n106 = Subtract(x=w88, y=w87) -> (x-y=w86:dbl)
            n107 = case shown="True" w79 {
              tunnel: w70 -> [w117 w121]
              tunnel: [w117 w120] -> w69
              tunnel: [FALSE ("stop") w118] -> w66
              frame False {
              }
              frame True {
                # "If the telemetry was started successfully the stroker Wizard is displayed \nif the current tool is Stroker, if not the dialog is closed"
                n108 = call "Selected Tool holder.vi"() -> ("Tool out"=w119:T46)  [unwired: 14 in, 1 out]
                n109 = case shown="\"Stroker\"" w119 {
                  tunnel: w121 -> [w123 w132]
                  tunnel: [w123 w131] -> w120
                  tunnel: [TRUE ("stop") FALSE ("stop")] -> w118
                  frame "Driller", Default {
                  }
                  frame "Stroker" {
                    n110 = local read "Size"() -> (w128:T2)
                    n111 = Not Equal?(x=w128, y=Slips_Type_Radio."No Selection" ("Size")) -> (x != y?=w127:bool)
                    n112 = property on="Property Node" class="VI"("Front Panel.Closeable"=w127) -> ()  [unwired: 2 in, 2 out]
                    n113 = property on="Tab Control" class="TabCtl (strict)"(error in=w132, "Value"=enum32{"Waiting", "Wizard", "Timeout"}."Wizard" ("Tab Control")) -> (error out=w131:errorcluster)  [unwired: 1 in, 1 out]
                    n114 = Select(t=T10."Enabled" ("Disabled"), s=w127, f=T10."Disabled and Grayed Out" ("Disabled")) -> (s? t:f=w124:T10)
                    n115 = property on="Close" class="Bool (strict)"("DisabledEnum"=w124) -> ()  [unwired: 2 in, 2 out]
                  }
                }
              }
            }
            n116 = Greater?(x=w86, y=w73) -> (0:w76:bool)
            n117 = Rotate 1D Array(1:w82, 2:1 ("n")) -> (0:w83:bool[])
            n118 = Array To Cluster(array=w83) -> (cluster=→"Waiting Lights":T47)
            n119 = Or(x=w81, y=w80) -> (x .or. y?=w77:bool)
            n120 = Compound Arithmetic op=AND(invert w77, w76, invert w75) -> (w78:bool)
            n121 = case shown="True" w78 {
              tunnel: w69 -> [w109 w114]
              tunnel: [w109 w111] -> w68
              frame False {
              }
              frame True {
                # "The telemetry CMD button is reset"
                n122 = property on="Property Node" class="VI"("Front Panel.Closeable"=TRUE ("Front Panel Window:Closeable")) -> ()  [unwired: 2 in, 2 out]
                n123 = property on="Tab Control" class="TabCtl (strict)"(error in=w114, "Value"=enum32{"Waiting", "Wizard", "Timeout"}."Timeout" ("Tab Control")) -> (error out=w112:errorcluster)  [unwired: 1 in, 1 out]
                n124 = call "QSM enque.vi"("State"=QSM_State_List."Reset Telemetry", "error in"=w112) -> ("error out"=w111:errorcluster)  [unwired: 13 in]
              }
            }
            n125 = Bundle By Name(cluster=w105, "Waiting lights"=w83, "Timed out"=w76, "Tool Connected"=w77) -> (w106:T45)
            n126 = call "emi_Wait until MS multipl with Err.vi"("millisecond multiple(0)"=u32 100, "error in (no error)"=w68) -> ("error out"=w107:errorcluster)  [unwired: 13 in]
          }
          frame "Stop" {
            # "To alow VI to exit befor \nAplicatin End.\nFor use in dialogs"
            # "Stop the loop. May be restarted later. Close interfaces and the like"
          }
          frame "Error Handling" {
            # "Loop automaticaly returns here after error is found. If error is cleared, \nLoop wil continue as normal(if was operative when error."
          }
          frame "End" {
            # "Only executes at application end has. Should performa any action the loop \nneeds to finnish. Executes only once."
          }
          frame "Post" {
            # "Only exists to pas true to loop conditional without extra VI. DO Not edit"
          }
        }
      }
      n127 = Merge Errors(w30, w29) -> (w28:errorcluster)
    }
  }
  n128 = call "emi_Dialog End.vi"("error in"=w9) -> ("error out"=w8:errorcluster)  [unwired: 14 in]
  n129 = call <vilib>:"Clear Errors.vi"("error in (no error)"=w8) -> ()  [unwired: 6 in, 1 out]
